vi "Update Test Name.vi"(8 "error in":errorcluster, 10 "Show":bool, 11 "Base Software in":refnum<class "Base Software.lvclass">) -> (0 "error out":errorcluster, 3 "Base Software out":refnum<class "Base Software.lvclass">)   [LabVIEW 2019, in "Base Software.lvlib" / "Main.lvlib" / "Base Software.lvclass"]
uses:
  Project/Base Software.lvclass
  builds/Engine/Engine.lvlibp/Project/Engine.lvclass
  C:/Users/Public/Documents/Development/builds/Engine/Engine.lvlibp/Project/Engine.lvclass
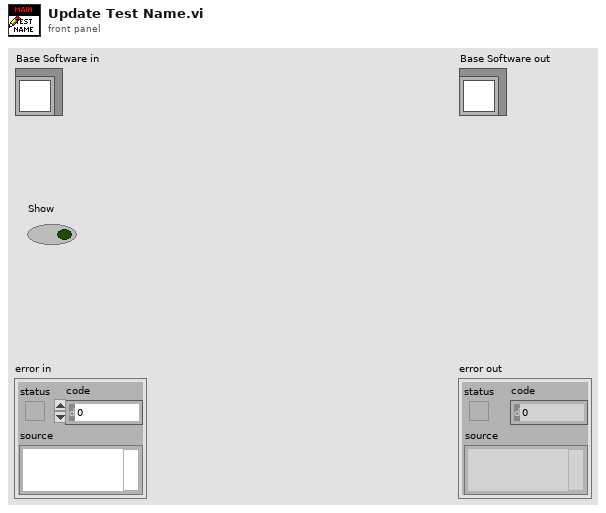
[diagram p1: front panel]
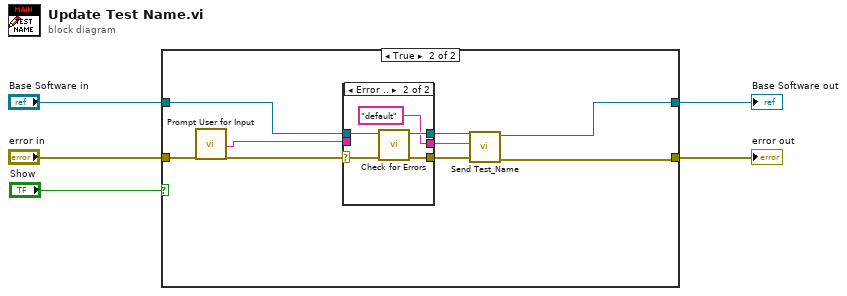
[diagram p0: block diagram]
diagram:
  n1 = case shown="True" "Show" {
    tunnel: "error in" -> [w6 w16]
    tunnel: "Base Software in" -> [w7 w15]
    tunnel: [w6 w9] -> w3
    tunnel: [w7 w10] -> w1
    frame False {
    }
    frame True {
      n2 = call "Prompt User for Input"("error in (no error)"=w16) -> ("Test Name"=w14:string, "error out"=w13:errorcluster)  [unwired: 16 in, 1 out]
      n3 = case shown="Error .." w13 {
        selector: w13 -> [w18 w23]
        tunnel: w15 -> [w19 w24]
        tunnel: [w19 w21] -> w11
        tunnel: [w18 w22] -> w12
        tunnel: w14 -> [w17 _]
        tunnel: [w17 "default"] -> w8
        frame No Error {
        }
        frame Error {
          n4 = call "Check for Errors.vi"("error in"=w23, "Engine in"=w24) -> ("error out"=w22:errorcluster, "Engine out"=w21:refnum<class "Base Software.lvclass">)  [unwired: 8 in]
        }
      }
      n5 = call "Send Test_Name.vi"("error in"=w12, "Test Name"=w8, "Engine in"=w11) -> ("error out"=w9:errorcluster, "Engine out"=w10:refnum<class "Base Software.lvclass">)  [unwired: 7 in]
    }
  }
  "error out" <- w3
  "Base Software out" <- w1
